vi "AutonomousTurn.vi"(10 "Speed":dbl format="%#_13g", 11 "Turn":dbl format="%#_13g") -> ()   [LabVIEW 2014]
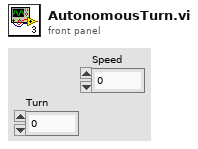
[diagram p1: front panel]
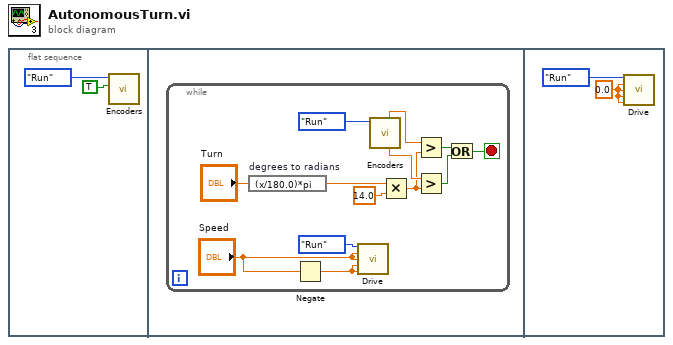
[diagram p0: block diagram]
diagram:
  n1 = flat-sequence {
    frame #0 {
      n2 = call "Encoders.vi"("Reset"=TRUE, "Enum"=enum16{"Start", "Run", "End"}."Run") -> ()  [unwired: 4 in, 6 out]
    }
    frame #1 {
      n3 = while {
        stop <- w9 stop-if-true
        n4 = expression code="(x/180.0)*pi" "degrees to radians"("Turn") -> (w5:dbl)
        n5 = Negate(x="Speed") -> (-x=w7:dbl)
        n6 = call "Drive.vi"("Enum"=enum16{"Start", "Run", "End"}."Run", "Left Primary"="Speed", "Left Secondary"="Speed", "Right Primary"=w7, "Right Secondary"=w7) -> ()  [unwired: 11 in]
        n7 = call "Encoders.vi"("Enum"=enum16{"Start", "Run", "End"}."Run") -> ("LDistance"=w12:dbl, "RDistance"=w13:dbl)  [unwired: 5 in, 4 out]
        n8 = Multiply(x=w5, y=14.0) -> (x*y=w3:dbl)
        n9 = Greater?(x=w13, y=w3) -> (0:w11:bool)
        n10 = Greater?(x=w12, y=w3) -> (0:w10:bool)
        n11 = Or(x=w11, y=w10) -> (x .or. y?=w9:bool)
      }
    }
    frame #2 {
      w16 = 0.0
      n12 = call "Drive.vi"("Enum"=enum16{"Start", "Run", "End"}."Run", "Left Primary"=w16, "Left Secondary"=w16, "Right Primary"=w16, "Right Secondary"=w16) -> ()  [unwired: 11 in]
    }
  }
